vi "MaiTaiEOMGUI.vi"() -> ()   [LabVIEW 2011]
panel:
  in  "laser mW":cluster{dbl, dbl}(slide) scale=10.0..1400.0
  in  "Wavelength":cluster{u16, u16}(slide)={750, 750} scale=700.0..990.0
  out "Maitai W":dbl
  in  "Log":bool
  in  "stop":bool
  in  "close":bool caption="Shutter"
  in  "off":bool caption="Laser"
  # "~1/2 @sample"
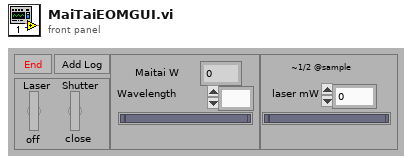
[diagram p1: front panel]
types:
  T1 = enum16{"None/#Datasets", "Clear", "TagValueOf#", "AddValues", "ReadValue", "ChangeValue", "Get all"}
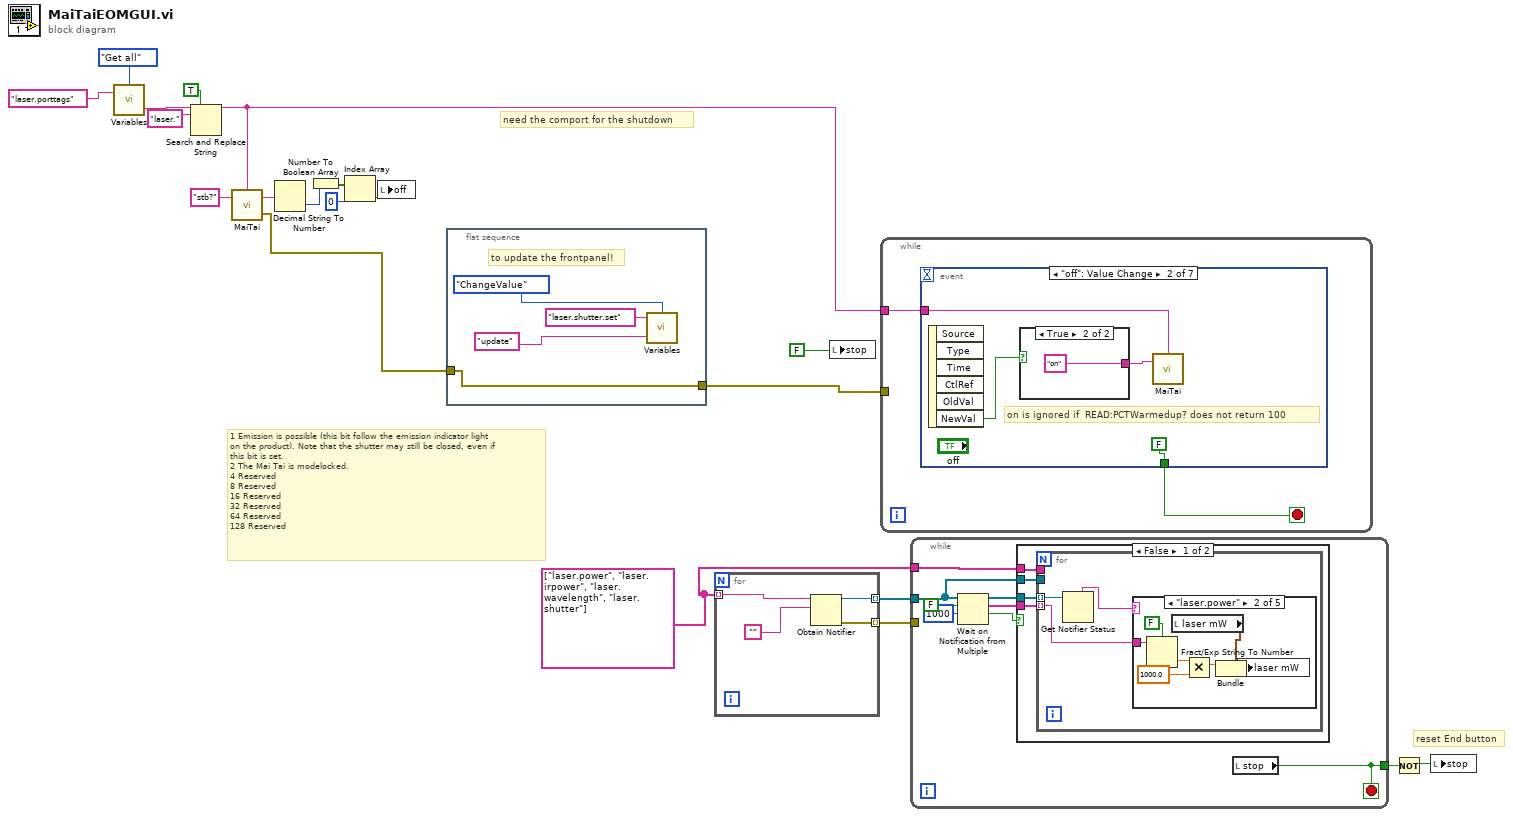
[diagram p0: block diagram]
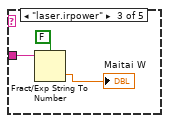
[diagram p3: hidden frame]
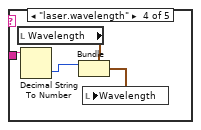
[diagram p4: hidden frame]
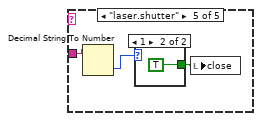
[diagram p5: hidden frame]
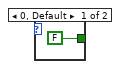
[diagram p6: hidden frame]
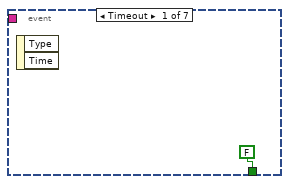
[diagram p8: hidden frame]
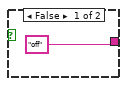
[diagram p9: hidden frame]
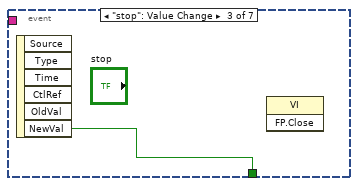
[diagram p10: hidden frame]
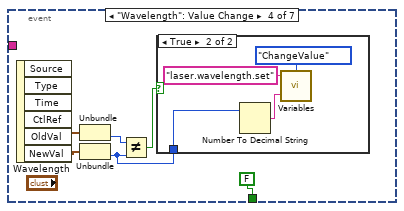
[diagram p11: hidden frame]
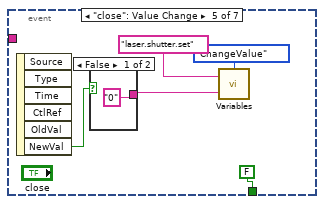
[diagram p13: hidden frame]
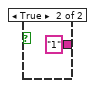
[diagram p14: hidden frame]
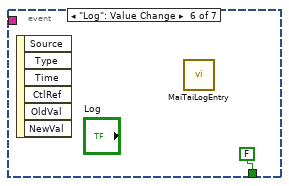
[diagram p15: hidden frame]
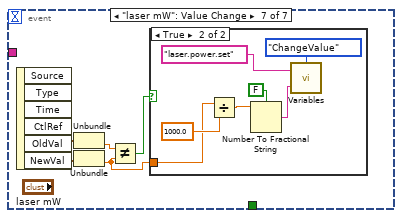
[diagram p16: hidden frame]
diagram:
  w6 = string[] ["laser.power", "laser.irpower", "laser.wavelength", "laser.shutter"]
  # "need the comport for the shutdown"
  # "reset End button"
  # "1 Emission is possible (this bit follow the emission indicator light\non the product). Note that the shutter may still be closed, even if\nthis bit is set.\n2 The Mai Tai is modelocked.\n4 Reserved\n8 Reserved\n16 Reserved\n32 Reserved\n64 Reserved\n128 Reserved"
  n1 = call "Variables.vi"("Tag in"="laser.porttags", "Command"=T1."Get all") -> ("value out"=w13:string)  [unwired: 1 in, 2 out]
  n2 = Search and Replace String(replace all?=TRUE ("replace all? (F)"), input string=w13, search string="laser.") -> (result string=w9:string)  [unwired: 1 in, 7 out]
  n3 = call "MaiTai.vi"("command"="stb?", "com parameters"=w9) -> ("error out"=w3:errorcluster, "read"=w19:string)  [unwired: 1 in, 1 out]
  n4 = Decimal String To Number(string=w19) -> (number=w10:i32)  [unwired: 3 out]
  n5 = Number To Boolean Array(number=w10) -> (Boolean array=w18:bool[])
  n6 = Index Array(array=w18, index=0) -> (element=w17:bool)
  n7 = local write "off"(w17) -> ()
  n8 = flat-sequence {
    tunnel: w3 -> [w24]
    tunnel: [w24] -> w2
    frame #0 {
      # "to update the frontpanel!"
      n9 = call "Variables.vi"("value"="update", "Tag in"="laser.shutter.set" ("Name"), "Command"=T1."ChangeValue") -> ()  [unwired: 1 in, 2 out]
    }
  }
  n10 = for {
    tunnel: [w27] -> w8 mode=indexing
    tunnel: [w26] -> w7 mode=indexing
    tunnel: w6 -> [w25] mode=indexing
    n11 = Obtain Notifier(name (unnamed)=w25, notification data type="") -> (notifier out=w26:refnum<notifier>, error out=w27:errorcluster)  [unwired: 2 in, 1 out]
  }
  n12 = local write "stop"(FALSE ("stop")) -> ()
  n13 = while {
    tunnel: w2 -> [_]
    tunnel: w9 -> [w29]
    stop <- w30 stop-if-true
    n14 = event shown="[1] \"off\": Value Change" {
      selector: _ -> [_ _ _ _ _ _ _]
      dyn-events: _ -> [_ _ _ _ _ _ _]
      timeout: _ -> [_ _ _ _ _ _ _]
      tunnel: [FALSE ("stop") FALSE ("stop") w38 FALSE ("stop") FALSE ("stop") FALSE ("stop") _] -> w30
      tunnel: w29 -> [_ w32 _ _ _ _ _]
      event Timeout {
        n15 = event-data() -> ()  [unwired: 3 out]
      }
      event "off": Value Change {
        # "on is ignored if  READ:PCTWarmedup? does not return 100"
        n16 = event-data() -> ("NewVal"=w35:bool)  [unwired: 6 out]
        n17 = case shown="True" w35 {
          tunnel: ["off" "on"] -> w34
          frame False {
          }
          frame True {
          }
        }
        n18 = call "MaiTai.vi"("command"=w34, "com parameters"=w32) -> ()  [unwired: 1 in, 3 out]
      }
      event "stop": Value Change {
        n19 = event-data() -> ("NewVal"=w38:bool)  [unwired: 6 out]
        n20 = invoke class="VI" method="FP.Close"() -> ()  [unwired: 3 in, 3 out]
      }
      event "Wavelength": Value Change {
        n21 = event-data() -> ("OldVal"=w43:cluster{u16, u16}, "NewVal"=w42:cluster{u16, u16})  [unwired: 5 out]
        n22 = Unbundle(w43) -> (w41:u16)  [unwired: 1 out]
        n23 = Unbundle(w42) -> (w39:u16)  [unwired: 1 out]
        n24 = Not Equal?(x=w41, y=w39) -> (x != y?=w40:bool)
        n25 = case shown="True" w40 {
          tunnel: w39 -> [_ w45]
          frame False {
            # "moved the indicator"
          }
          frame True {
            n26 = Number To Decimal String(number=w45) -> (decimal integer string=w47:string)  [unwired: 1 out]
            n27 = call "Variables.vi"("value"=w47, "Tag in"="laser.wavelength.set" ("Name"), "Command"=T1."ChangeValue") -> ()  [unwired: 1 in, 2 out]
          }
        }
      }
      event "close": Value Change {
        n28 = event-data() -> ("NewVal"=w53:bool)  [unwired: 6 out]
        n29 = case shown="False" w53 {
          tunnel: ["0" "1"] -> w49
          frame False {
          }
          frame True {
          }
        }
        n30 = call "Variables.vi"("value"=w49, "Tag in"="laser.shutter.set" ("Name"), "Command"=T1."ChangeValue") -> ()  [unwired: 1 in, 2 out]
      }
      event "Log": Value Change {
        n31 = event-data() -> ()  [unwired: 7 out]
        n32 = call "MaiTaiLogEntry.vi"() -> ()  [unwired: 1 out]
      }
      event "laser mW": Value Change {
        n33 = event-data() -> ("OldVal"=w61:cluster{dbl, dbl}, "NewVal"=w60:cluster{dbl, dbl})  [unwired: 5 out]
        n34 = Unbundle(w61) -> (w59:dbl)  [unwired: 1 out]
        n35 = Unbundle(w60) -> (w57:dbl)  [unwired: 1 out]
        n36 = Not Equal?(x=w59, y=w57) -> (x != y?=w58:bool)
        n37 = case shown="True" w58 {
          tunnel: w57 -> [_ w62]
          frame False {
          }
          frame True {
            n38 = Divide(x=w62, y=1000.0) -> (x/y=w67:dbl)
            n39 = Number To Fractional String(use system decimal point (T)=FALSE, number=w67) -> (F-format string=w64:string)  [unwired: 2 out]
            n40 = call "Variables.vi"("value"=w64, "Tag in"="laser.power.set" ("Name"), "Command"=T1."ChangeValue") -> ()  [unwired: 1 in, 2 out]
          }
        }
      }
    }
  }
  n41 = while {
    tunnel: w7 -> [w71]
    tunnel: w8 -> [_]
    tunnel: w6 -> [w70]
    tunnel: [w69] -> w4
    stop <- w69 stop-if-true
    n42 = Wait on Notification from Multiple(0:w71, 1:FALSE ("ignore previous (F)"), 2:1000 ("timeout in ms (-1)")) -> (8:w75:refnum<notifier>[], 9:w76:string[], 10:w74:bool)  [unwired: 1 in, 1 out]
    n43 = case shown="False" w74 {
      tunnel: w76 -> [w77 _]
      tunnel: w75 -> [w80 _]
      tunnel: w71 -> [w79 _]
      tunnel: w70 -> [w78 _]
      frame False {
        n44 = for {
          tunnel: w80 -> [w82] mode=indexing
          tunnel: w79 -> [_]
          tunnel: w78 -> [_]
          tunnel: w77 -> [w83] mode=indexing
          n45 = Get Notifier Status(notifier=w82) -> (notifier name=w81:string)  [unwired: 1 in, 4 out]
          n46 = case shown="\"laser.power\"" w81 {
            tunnel: w83 -> [_ w87 w92 w97 w98]
            frame "False", Default {
              # "nothing"
            }
            frame "laser.power" {
              n47 = Fract/Exp String To Number(use system decimal point (T)=FALSE, string=w87) -> (number=w89:dbl)  [unwired: 3 out]
              n48 = local read "laser mW"() -> (w85:cluster{dbl, dbl})
              n49 = Multiply(x=w89, y=1000.0) -> (x*y=w86:dbl)
              n50 = Bundle(cluster=w85, w86) -> (w84:cluster{dbl, dbl})  [unwired: 1 out]
              n51 = local write "laser mW"(w84) -> ()
            }
            frame "laser.irpower" {
              n52 = Fract/Exp String To Number(use system decimal point (T)=FALSE, string=w92) -> (number=→"Maitai W":dbl)  [unwired: 3 out]
            }
            frame "laser.wavelength" {
              n53 = local read "Wavelength"() -> (w96:cluster{u16, u16})
              n54 = Decimal String To Number(string=w97) -> (number=w95:i32)  [unwired: 3 out]
              n55 = Bundle(cluster=w96, w95) -> (w94:cluster{u16, u16})  [unwired: 1 out]
              n56 = local write "Wavelength"(w94) -> ()
            }
            frame "laser.shutter" {
              n57 = Decimal String To Number(string=w98) -> (number=w100:i32)  [unwired: 3 out]
              n58 = case shown="1" w100 {
                tunnel: [FALSE TRUE] -> w99
                frame 0, Default {
                }
                frame 1 {
                }
              }
              n59 = local write "close"(w99) -> ()
            }
          }
        }
      }
      frame True {
        # "to check stop"
      }
    }
    n60 = local read "stop"() -> (w69:bool)
  }
  n61 = Not(x=w4) -> (.not. x?=w5:bool)
  n62 = local write "stop"(w5) -> ()
